vi "P2022 TB INCAR_Initialize.vi"(8 "error in (no error)":errorcluster, 11 "User event":T4) -> (0 "error out":errorcluster, 1 "FLOWBUS_MassFlows":T1={"Dispositivos"=[["3", "NO", "M0000013", "Air", "10", "ln/mn", "0", "0"], ["4", "NO", "M0000014", "Air", "10", "ln/mn", "0", "0"], ["5", "NO", "M0000015", "Air", "10", "ln/mn", "0", "0"], ["6", "NO", "M0000016", "Air", "10", "ln/mn", "0", "0"], ["7", "NO", "M0000017", "Air", "10", "ln/mn", "0", "0"], ["8", "NO", "M0000018", "Air", "10", "ln/mn", "0", "0"]], "NuevosSP"=[["0", "NO", "M0000013", "Air", "1", "ln/mn", "0", "0"], ["0", "NO", "M0000014", "Air", "1", "ln/mn", "0", "0"], ["0", "NO", "M0000015", "Air", "1", "ln/mn", "0", "0"], ["0", "NO", "M0000016", "Air", "1", "ln/mn", "0", "0"], ["0", "NO", "M0000017", "Air", "1", "ln/mn", "0", "0"], ["0", "NO", "M0000018", "Air", "1", "ln/mn", "0", "0"]], "Nodes"=4, "Delay(s)"=0.075}, 2 "SERIAL_MassFlows":T1={"Dispositivos"=[["3", "NO", "M0000013", "Air", "10", "ln/mn", "0", "0"], ["4", "NO", "M0000014", "Air", "10", "ln/mn", "0", "0"], ["5", "NO", "M0000015", "Air", "10", "ln/mn", "0", "0"], ["6", "NO", "M0000016", "Air", "10", "ln/mn", "0", "0"], ["7", "NO", "M0000017", "Air", "10", "ln/mn", "0", "0"], ["8", "NO", "M0000018", "Air", "10", "ln/mn", "0", "0"]], "NuevosSP"=[["0", "NO", "M0000013", "Air", "1", "ln/mn", "0", "0"], ["0", "NO", "M0000014", "Air", "1", "ln/mn", "0", "0"], ["0", "NO", "M0000015", "Air", "1", "ln/mn", "0", "0"], ["0", "NO", "M0000016", "Air", "1", "ln/mn", "0", "0"], ["0", "NO", "M0000017", "Air", "1", "ln/mn", "0", "0"], ["0", "NO", "M0000018", "Air", "1", "ln/mn", "0", "0"]], "Nodes"=4, "Delay(s)"=0.075}, 3 "Comunicaciones":T3={"Flujo_1"="ASRL6::INSTR", "Brk1"=FALSE, "Flujo_2"="ASRL6::INSTR", "Brk2"=FALSE, "Flujo_3"="ASRL6::INSTR", "Brk3"=FALSE, "Flujo_4"="ASRL6::INSTR", "Brk4"=FALSE, "Eurothe"="ASRL6::INSTR", "Eurot"=FALSE, "Balanza"="ASRL6::INSTR", "Bal"=FALSE, "eValPos"="ASRL6::INSTR", "eVal"=FALSE, "flowbus"="ASRL6::INSTR", "fb"=FALSE})   [LabVIEW 2013]
uses:
  Controles/User Event Reference.ctl
  Controles/User Event Data.ctl
  Controles/Data Type.ctl
  Controles/P2018 Com Control.ctl
  Controles/P2018 Bronkhorst Control.ctl
  serialBronkhorst/_s_TablaBronkhorst.ctl
  Display/Display_Command Control.ctl
  serialTermobDisbal/Multicard III_Hardware_Module Control.ctl
  serialArduinoMicro/ArduinoMicro Module Control.ctl
  P2022 TB INCAR GLOBALES.vi
  modbusEurotherm P116_485/Eurotherm_Hardware_Module Control.ctl
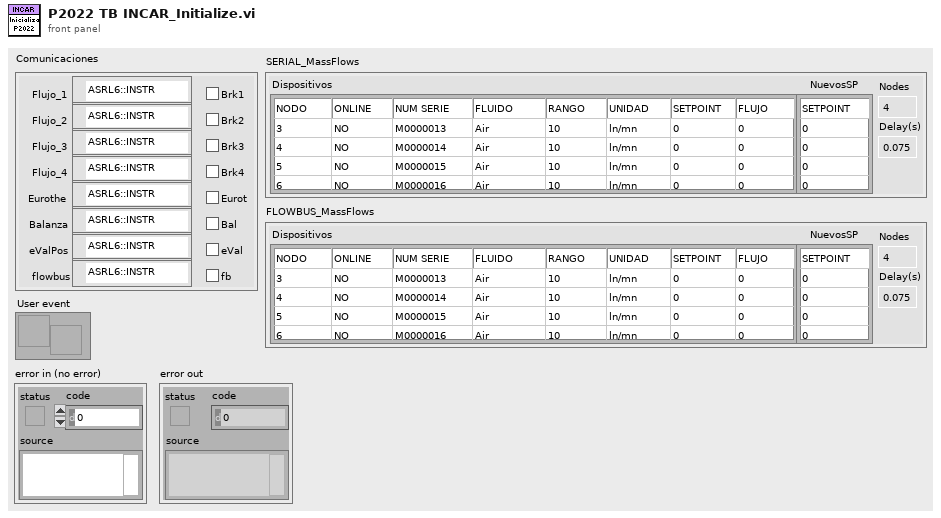
[diagram p1: front panel]
types:
  T1 = typedef "P2018 Bronkhorst Control.ctl" = cluster{"Dispositivos":T2, "NuevosSP":string[][], "Nodes":u32, "Delay(s)":dbl}
  T2 = typedef "_s_TablaBronkhorst.ctl" = string[][]
  T3 = typedef "P2018 Com Control.ctl" = cluster{"Flujo_1":refnum<visa-resource-name>, "Brk1":bool, "Flujo_2":refnum<visa-resource-name>, "Brk2":bool, "Flujo_3":refnum<visa-resource-name>, "Brk3":bool, "Flujo_4":refnum<visa-resource-name>, "Brk4":bool, "Eurothe":refnum<visa-resource-name>, "Eurot":bool, "Balanza":refnum<visa-resource-name>, "Bal":bool, "eValPos":refnum<visa-resource-name>, "eVal":bool, "flowbus":refnum<visa-resource-name>, "fb":bool}
  T4 = typedef "User Event Reference.ctl" = refnum<user-event>
  T5 = typedef "ArduinoMicro Module Control.ctl" = enum16{"Initialize", "Read Data", "Write Data", "Enable", "Disable", "Shutdown"}
  T6 = typedef "Multicard III_Hardware_Module Control.ctl" = enum16{"Initialize", "Cero", "Span", "Read ugr", "Read mgr", "Read A/D", "Read T", "Number readings", "Thermocouple type", "Status", "Shutdown"}
  T7 = typedef "Data Type.ctl" = enum16{"Init FP", "En/Dis FP Ctls", "Update FP", "Upd Status", "Upd Seq"}
  T8 = typedef "Display_Command Control.ctl" = enum16{"Initialize", "Generate Event", "Shutdown"}
  T9 = typedef "Eurotherm_Hardware_Module Control.ctl" = enum16{"Initialize", "Write SP", "Read SP+PV", "Write Rate", "Set P", "Set I", "Set D", "Shutdown"}
  T10 = typedef "_f_TablaBronkhorst.ctl" = string[][]
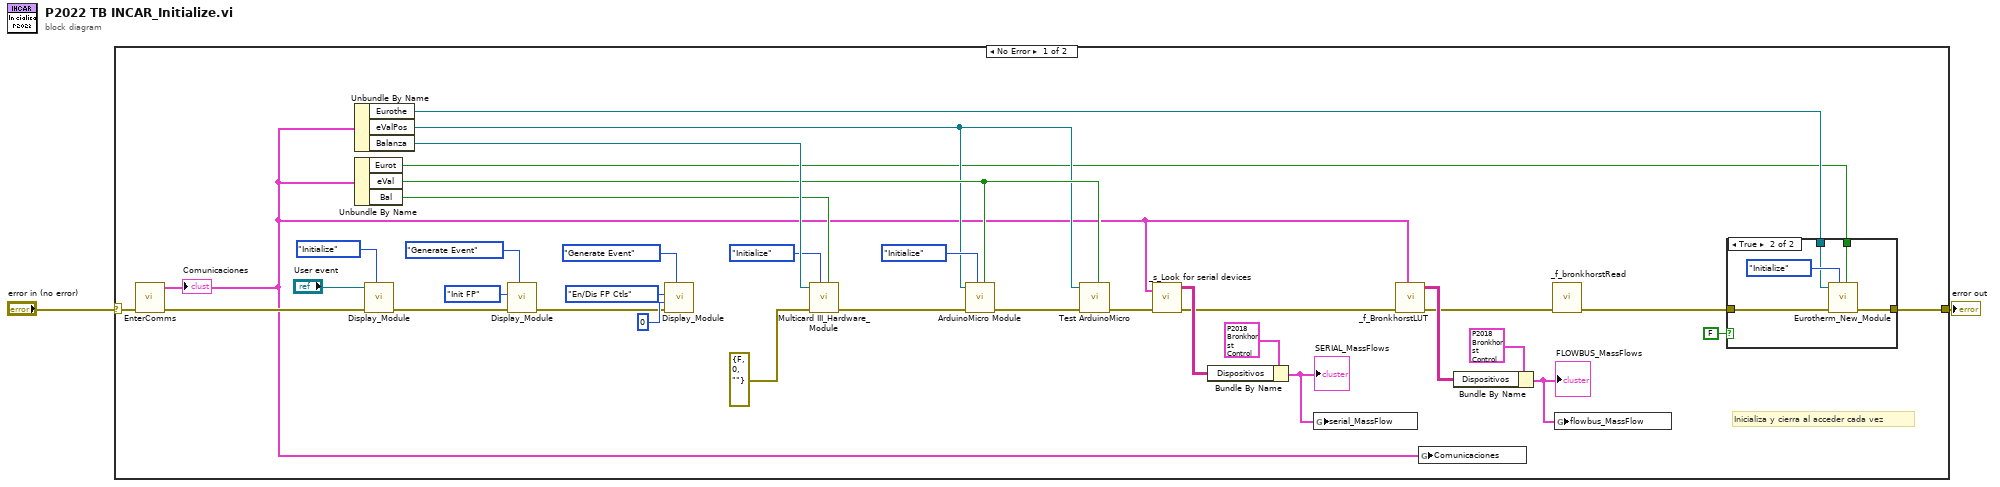
[diagram p0: block diagram]
diagram:
  n1 = case shown="No Error" "error in (no error)" {
    selector: "error in (no error)" -> [w33 w44]
    tunnel: [w18 w44] -> w1
    frame No Error {
      # "Inicializa y cierra al acceder cada vez"
      n2 = call "EnterComms.vi"("error in (no error)"=w33) -> ("error out"=w23:errorcluster, "Comunicaciones"=w10:T3)  [unwired: 8 in, 1 out]
      "Comunicaciones" <- w10
      n3 = Unbundle By Name(w10) -> ("Eurothe"=w17:refnum<visa-resource-name>, "eValPos"=w19:refnum<visa-resource-name>, "Balanza"=w27:refnum<visa-resource-name>)
      n4 = Unbundle By Name(w10) -> ("Eurot"=w16:bool, "eVal"=w20:bool, "Bal"=w15:bool)
      n5 = call "Display_Module.vi"("Command"=Display_Command_Control."Initialize", "error in (no error)"=w23, "user event out"="User event") -> ("error out"=w35:errorcluster)  [unwired: 8 in]
      n6 = call "Display_Module.vi"("Command"=Display_Command_Control."Generate Event", "error in (no error)"=w35, "Data Type"=Data_Type."Init FP") -> ("error out"=w34:errorcluster)  [unwired: 8 in]
      n7 = call "Display_Module.vi"("Command"=Display_Command_Control."Generate Event", "error in (no error)"=w34, "Data"=0, "Data Type"=Data_Type."En/Dis FP Ctls") -> ()  [unwired: 7 in, 1 out]
      n8 = call "Multicard III_Hardware_Module.vi"("Multicard (T:Enable)"=w15, "Command"=Multicard_III_Hardware_Module_Control."Initialize", "error in (no error)"=errorcluster {"status"=FALSE, "code"=0, "source"=""}, "VISA resource name"=w27) -> ("error out"=w24:errorcluster)  [unwired: 4 in, 3 out]
      n9 = call "ArduinoMicro Module.vi"("Enable"=w20, "Command"=ArduinoMicro_Module_Control."Initialize", "error in (no error)"=w24, "VISA resource name"=w19) -> ("error out"=w22:errorcluster)  [unwired: 3 in, 4 out]
      n10 = call "Test ArduinoMicro.vi"("Enable"=w20, "error in"=w22, "VISA resource name"=w19) -> ("error out"=w21:errorcluster)  [unwired: 8 in]
      n11 = call "_s_Look for serial devices.vi"("Comunicaciones"=w10, "error in (no error)"=w21) -> ("error out"=w11:errorcluster, "Dispositivos"=w12:T2)  [unwired: 8 in]
      n12 = Bundle By Name(cluster=T1 {"Dispositivos"=[["3", "NO", "M0000013", "Air", "10", "ln/mn", "0", "0"], ["4", "NO", "M0000014", "Air", "10", "ln/mn", "0", "0"], ["5", "NO", "M0000015", "Air", "10", "ln/mn", "0", "0"], ["6", "NO", "M0000016", "Air", "10", "ln/mn", "0", "0"], ["7", "NO", "M0000017", "Air", "10", "ln/mn", "0", "0"], ["8", "NO", "M0000018", "Air", "10", "ln/mn", "0", "0"]], "NuevosSP"=[["0", "NO", "M0000013", "Air", "1", "ln/mn", "0", "0"], ["0", "NO", "M0000014", "Air", "1", "ln/mn", "0", "0"], ["0", "NO", "M0000015", "Air", "1", "ln/mn", "0", "0"], ["0", "NO", "M0000016", "Air", "1", "ln/mn", "0", "0"], ["0", "NO", "M0000017", "Air", "1", "ln/mn", "0", "0"], ["0", "NO", "M0000018", "Air", "1", "ln/mn", "0", "0"]], "Nodes"=4, "Delay(s)"=0.075} ("MassFlow"), "Dispositivos"=w12) -> (w7:T1)
      "SERIAL_MassFlows" <- w7
      n13 = global write "P2022 TB INCAR GLOBALES.vi" "serial_MassFlow"(w7) -> ()
      n14 = call "_f_BronkhorstLUT.vi"("Comunicaciones"=w10, "error in (no error)"=w11) -> ("error out"=w5:errorcluster, "Dispositivos"=w9:T10)  [unwired: 8 in]
      n15 = global write "P2022 TB INCAR GLOBALES.vi" "Comunicaciones"(w10) -> ()
      n16 = Bundle By Name(cluster=T1 {"Dispositivos"=[["3", "NO", "M0000013", "Air", "10", "ln/mn", "0", "0"], ["4", "NO", "M0000014", "Air", "10", "ln/mn", "0", "0"], ["5", "NO", "M0000015", "Air", "10", "ln/mn", "0", "0"], ["6", "NO", "M0000016", "Air", "10", "ln/mn", "0", "0"], ["7", "NO", "M0000017", "Air", "10", "ln/mn", "0", "0"], ["8", "NO", "M0000018", "Air", "10", "ln/mn", "0", "0"]], "NuevosSP"=[["0", "NO", "M0000013", "Air", "1", "ln/mn", "0", "0"], ["0", "NO", "M0000014", "Air", "1", "ln/mn", "0", "0"], ["0", "NO", "M0000015", "Air", "1", "ln/mn", "0", "0"], ["0", "NO", "M0000016", "Air", "1", "ln/mn", "0", "0"], ["0", "NO", "M0000017", "Air", "1", "ln/mn", "0", "0"], ["0", "NO", "M0000018", "Air", "1", "ln/mn", "0", "0"]], "Nodes"=4, "Delay(s)"=0.075} ("MassFlow"), "Dispositivos"=w9) -> (w6:T1)
      "FLOWBUS_MassFlows" <- w6
      n17 = call "_f_bronkhorstRead.vi"("error in (no error)"=w5) -> ("error out"=w4:errorcluster)  [unwired: 9 in, 1 out]
      n18 = global write "P2022 TB INCAR GLOBALES.vi" "flowbus_MassFlow"(w6) -> ()
      n19 = case shown="True" FALSE {
        tunnel: w4 -> [w38 w43]
        tunnel: [w38 w42] -> w18
        tunnel: w17 -> [_ w40]
        tunnel: w16 -> [_ w39]
        frame False {
        }
        frame True {
          n20 = call "Eurotherm_New_Module.vi"("Eurotherm (T:Enable)"=w39, "Command"=Eurotherm_Hardware_Module_Control."Initialize", "error in (no error)"=w43, "VISA resource name"=w40) -> ("error out"=w42:errorcluster)  [unwired: 6 in, 1 out]
        }
      }
    }
    frame Error {
    }
  }
  "error out" <- w1
